vi "Set Path.vi"(8 "error in (no error)":errorcluster, 10 "Path":path, 11 "WebProjectPanel in":refnum<class "WebProjectPanel.lvclass">) -> (0 "error out":errorcluster, 3 "WebProjectPanel out":refnum<class "WebProjectPanel.lvclass">)   [LabVIEW 2020, in "PicoG-Processor.lvlib" / "WebProjectPanel.lvclass"]
uses:
  WebProjectPanel.lvclass
  WebProjectPanel.lvclass/WebProjectPanel.ctl
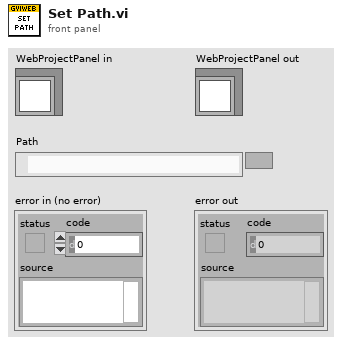
[diagram p1: front panel]
types:
  T1 = typedef "PicoG-Processor.lvlib/WebProjectPanel.lvclass/Ref Data.ctl" = cluster{"Last Update":dbl, "Path":path, "App Name":string, "Build Present":bool, "Deploy":refnum<user-event>}
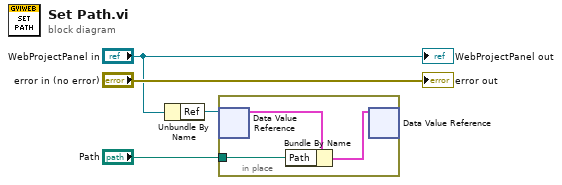
[diagram p0: block diagram]
diagram:
  n1 = Unbundle By Name("WebProjectPanel in") -> ("Ref"=w3:refnum<data-value>)
  n2 = in-place {
    in-place-border: "Path" -> [w5]
    n3 = in-place-dvr #1(w3) -> (w7:T1)  [unwired: 1 out]
    n4 = Bundle By Name(cluster=w7, "Path"=w5) -> (w6:T1)
    n5 = in-place-dvr #1(w6) -> ()  [unwired: 2 out]
  }
  "error out" <- "error in (no error)"
  "WebProjectPanel out" <- "WebProjectPanel in"
